vi "GTH.DAC.vi"(6 "FileName":string, 7 "CMD":T1(ring), 8 "Error In":errorcluster, 9 "AMP":u8=1 max=100 step=1, 10 "FREQ":u16, 11 "VISA_USB":refnum<visa-resource-name>) -> (0 "Error Out":errorcluster, 2 "Send CMD":string, 3 "OK?":bool)   [LabVIEW 2012, in "Lib_UEL.ATE.lvlib" / "STM32-CoreBD.lvlib"]
uses:
  STM32-CoreBD.lvlib
  <vilib>/regexp/Match Regular Expression.xnode
panel:
  # "Version History\nV01,2015-2-10, 初始版本."
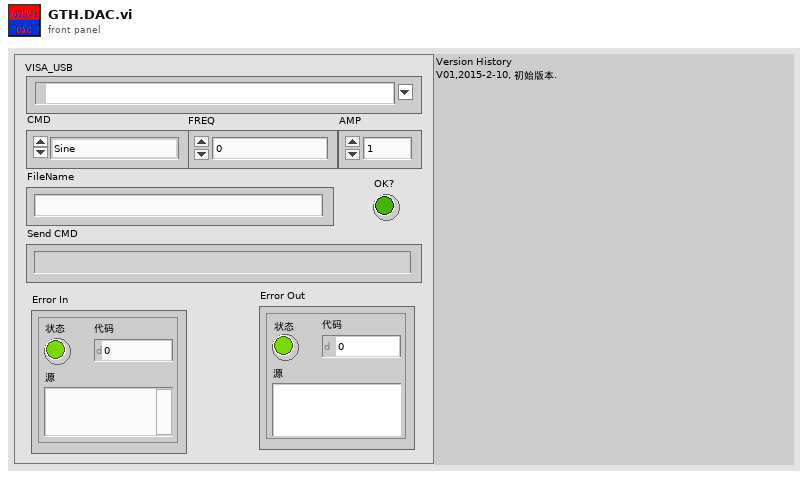
[diagram p1: front panel]
types:
  T1 = enum16{"Sine", "File", "ON_Chip_Pinknoise", "Close Output"}
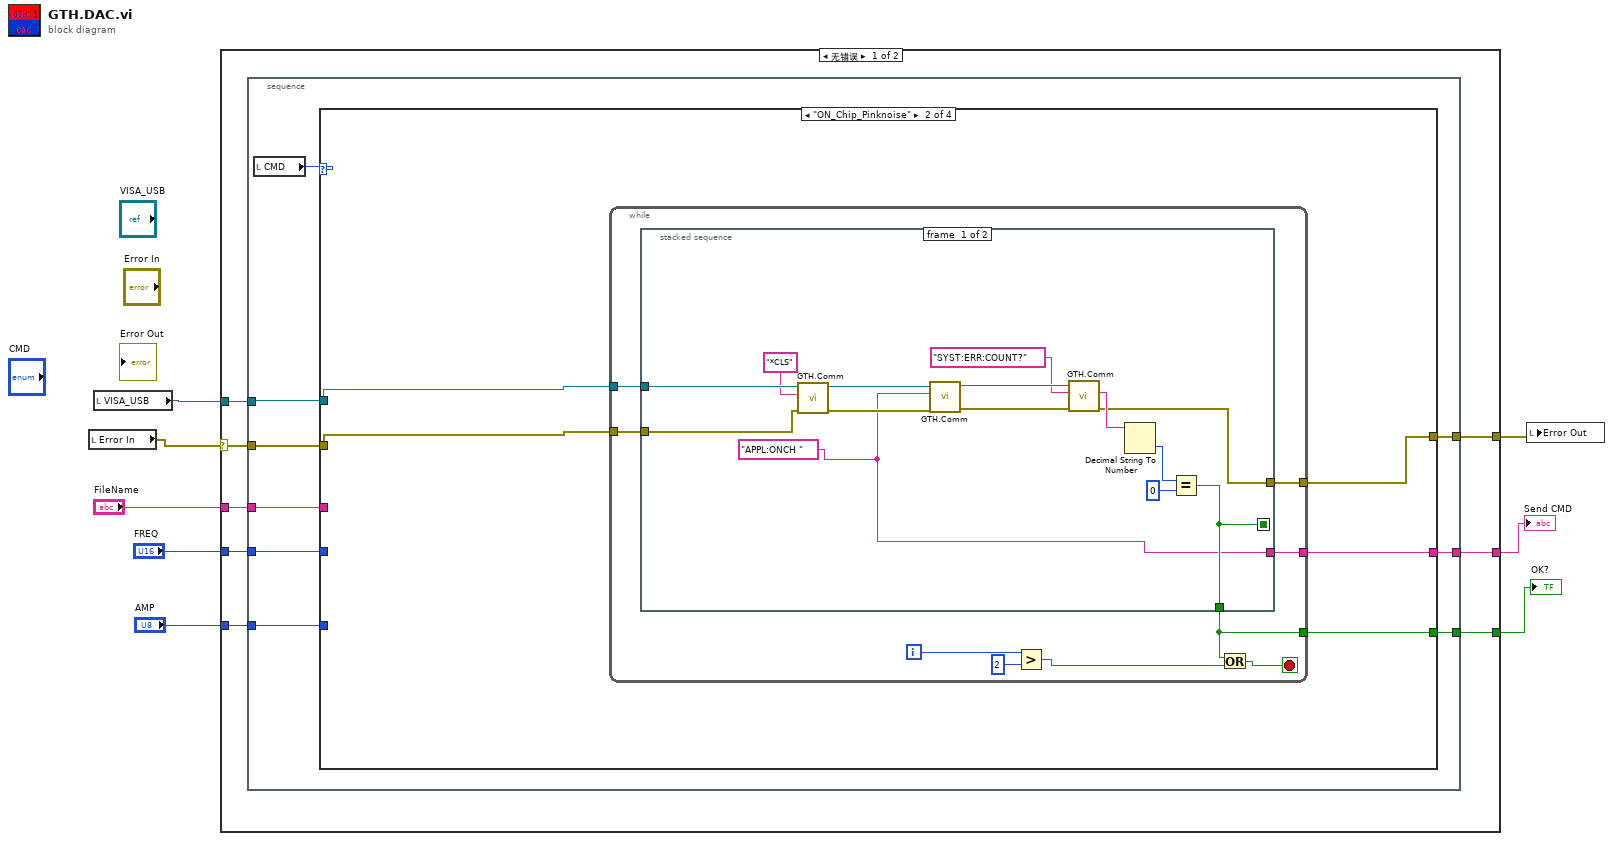
[diagram p0: block diagram]
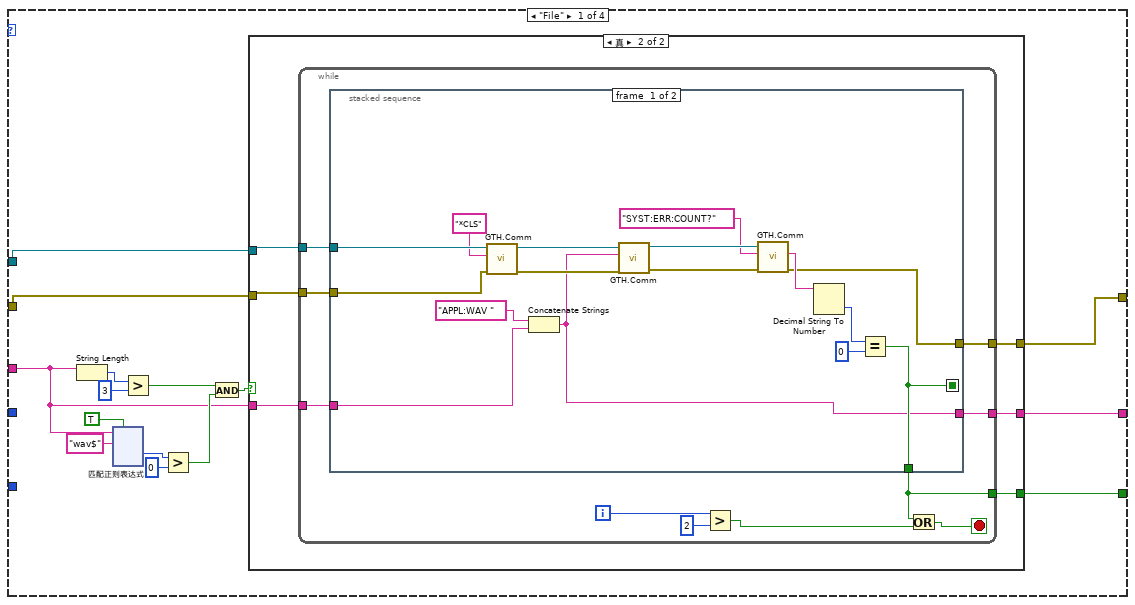
[diagram p2: hidden frame]
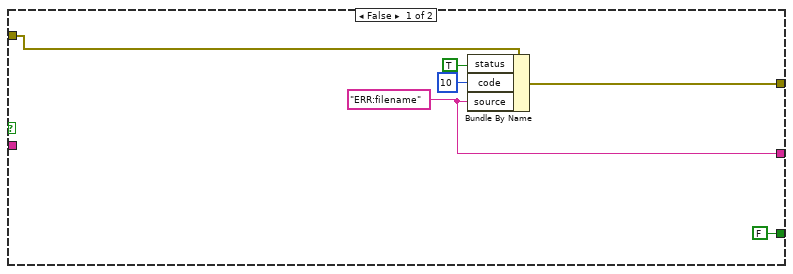
[diagram p3: hidden frame]
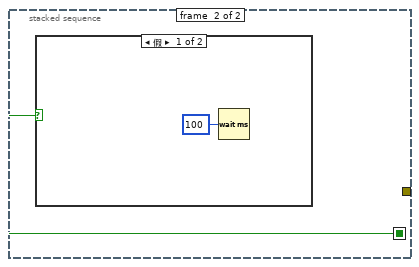
[diagram p4: hidden frame]
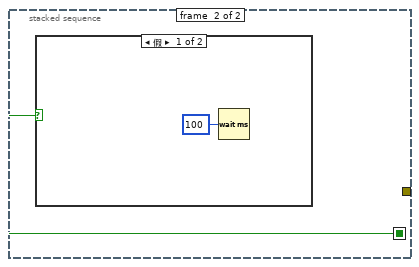
[diagram p6: hidden frame]
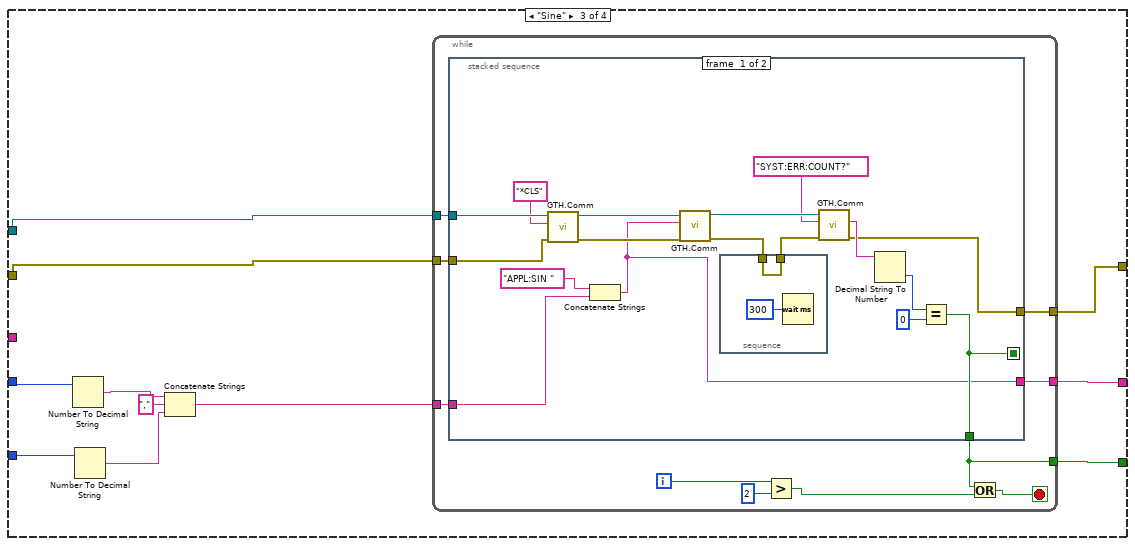
[diagram p8: hidden frame]
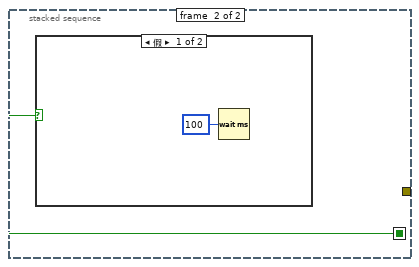
[diagram p9: hidden frame]
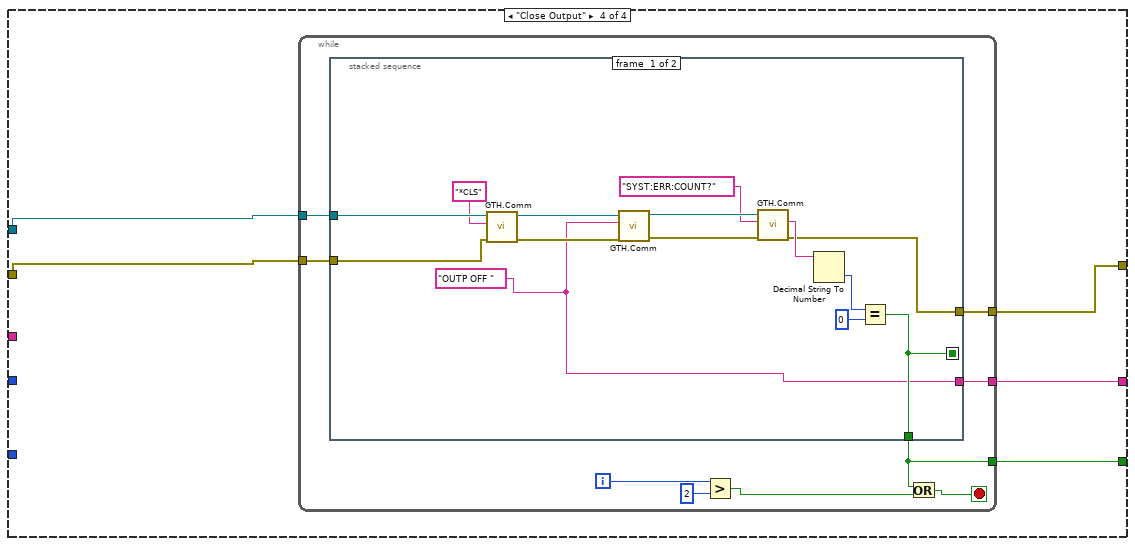
[diagram p11: hidden frame]
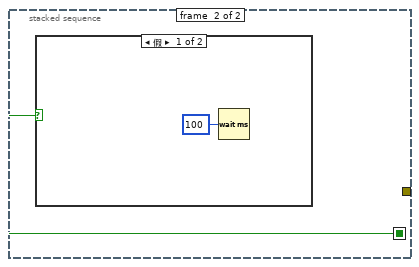
[diagram p12: hidden frame]
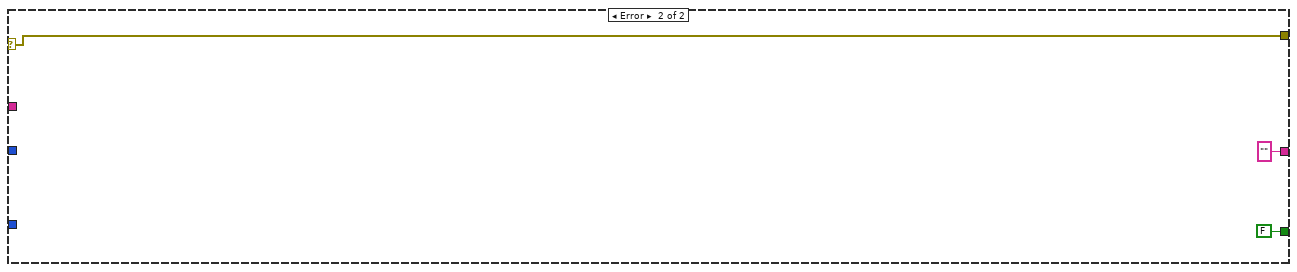
[diagram p14: hidden frame]
diagram:
  n1 = local read "Error In"() -> (w8:errorcluster)
  n2 = local read "VISA_USB"() -> (w6:refnum<visa-resource-name>)
  n3 = case shown="无错误" w8 {
    selector: w8 -> [w16 w296]
    tunnel: [w15 w296] -> w7
    tunnel: w6 -> [w14 _]
    tunnel: "FileName" -> [w13 _]
    tunnel: [w12 "" ("SCPI CMD")] -> w4
    tunnel: [w11 FALSE] -> w3
    tunnel: "FREQ" -> [w10 _]
    tunnel: "AMP" -> [w9 _]
    frame No Error {
      n4 = stacked-sequence {
        tunnel: w16 -> [w23]
        tunnel: [w22] -> w15
        tunnel: w14 -> [w24]
        tunnel: w13 -> [w21]
        tunnel: [w20] -> w12
        tunnel: [w19] -> w11
        tunnel: w10 -> [w18]
        tunnel: w9 -> [w17]
        frame #0 {
          n5 = local read "CMD"() -> (w25:T1)
          n6 = case shown="\"ON_Chip_Pinknoise\"" w25 {
            tunnel: w24 -> [w40 w196 w232 w268]
            tunnel: w23 -> [w39 w195 w231 w267]
            tunnel: [w29 w194 w230 w266] -> w22
            tunnel: w21 -> [w28 _ _ _]
            tunnel: [w27 w193 w229 w265] -> w20
            tunnel: [w26 w192 w228 w264] -> w19
            tunnel: w18 -> [_ _ w227 _]
            tunnel: w17 -> [_ _ w226 _]
            frame "File" {
              n7 = String Length(string=w28) -> (length=w38:i32)
              n8 = xnode "匹配正则表达式"("输入字符串"=w28, "正则表达式"="wav$", "忽略大小写？(F)"=TRUE) -> ("匹配后偏移量"=w34:i32)  [unwired: 3 in, 4 out]
              n9 = Greater?(x=w38, y=3) -> (0:w32:bool)
              n10 = Greater?(x=w34, y=0) -> (0:w31:bool)
              n11 = And(x=w32, y=w31) -> (x .and. y?=w30:bool)
              n12 = case shown="真" w30 {
                tunnel: w40 -> [_ w52]
                tunnel: w39 -> [w46 w51]
                tunnel: [w45 w49] -> w29
                tunnel: w28 -> [_ w50]
                tunnel: [w42 w48] -> w27
                tunnel: [FALSE w47] -> w26
                frame False {
                  w42 = "ERR:filename" ("source")
                  n13 = Bundle By Name(cluster=w46, "status"=TRUE, "code"=10, "source"=w42) -> (w45:errorcluster)
                }
                frame True {
                  n14 = while {
                    tunnel: w52 -> [w62]
                    tunnel: w51 -> [w61]
                    tunnel: w50 -> [w60]
                    tunnel: [w59] -> w49
                    tunnel: [w54] -> w48
                    tunnel: [w53] -> w47
                    i -> [w57]
                    stop <- w58 stop-if-true
                    n15 = stacked-sequence {
                      seq-local: [w64 _] -> [_ w79]
                      tunnel: w62 -> [w78 _]
                      tunnel: w61 -> [w77 _]
                      tunnel: w60 -> [w72 _]
                      tunnel: [w67 _] -> w59
                      tunnel: [w64 _] -> w53
                      tunnel: [w63 _] -> w54
                      frame #0 {
                        n16 = call "GTH.Comm.vi"("Error In"=w77, "SCPI CMD"="*CLS", "USB Port In"=w78) -> ("Error Out"=w74:errorcluster, "USB Port Out"=w75:refnum<visa-resource-name>)  [unwired: 3 in, 4 out]
                        n17 = Concatenate Strings("APPL:WAV " ("SCPI CMD"), w72) -> (w63:string)
                        n18 = call "GTH.Comm.vi"("Error In"=w74, "SCPI CMD"=w63, "USB Port In"=w75) -> ("Error Out"=w70:errorcluster, "USB Port Out"=w71:refnum<visa-resource-name>)  [unwired: 3 in, 4 out]
                        n19 = call "GTH.Comm.vi"("Error In"=w70, "SCPI CMD"="SYST:ERR:COUNT?", "USB Port In"=w71) -> ("Error Out"=w67:errorcluster, "Return"=w68:string)  [unwired: 3 in, 4 out]
                        n20 = Decimal String To Number(string=w68) -> (number=w66:i32)  [unwired: 2 in, 1 out]
                        n21 = Equal?(x=w66, y=0) -> (x = y?=w64:bool)
                      }
                      frame #1 {
                        n22 = case shown="假" w79 {
                          frame False {
                            n23 = Wait (ms)(milliseconds to wait=u32 100 ("等待时间（毫秒）")) -> ()  [unwired: 1 out]
                          }
                          frame True {
                          }
                        }
                      }
                    }
                    n24 = Greater?(x=w57, y=2) -> (0:w55:bool)
                    n25 = Or(x=w53, y=w55) -> (x .or. y?=w58:bool)
                  }
                }
              }
            }
            frame "ON_Chip_Pinknoise" {
              n26 = while {
                tunnel: w196 -> [w205]
                tunnel: w195 -> [w204]
                tunnel: [w203] -> w194
                tunnel: [w198] -> w193
                tunnel: [w197] -> w192
                i -> [w201]
                stop <- w202 stop-if-true
                n27 = stacked-sequence {
                  seq-local: [w207 _] -> [_ w220]
                  tunnel: w205 -> [w219 _]
                  tunnel: w204 -> [w218 _]
                  tunnel: [w210 _] -> w203
                  tunnel: [w207 _] -> w197
                  tunnel: [w206 _] -> w198
                  frame #0 {
                    w206 = "APPL:ONCH " ("SCPI CMD")
                    n28 = call "GTH.Comm.vi"("Error In"=w218, "SCPI CMD"="*CLS", "USB Port In"=w219) -> ("Error Out"=w215:errorcluster, "USB Port Out"=w216:refnum<visa-resource-name>)  [unwired: 3 in, 4 out]
                    n29 = call "GTH.Comm.vi"("Error In"=w215, "SCPI CMD"=w206, "USB Port In"=w216) -> ("Error Out"=w213:errorcluster, "USB Port Out"=w214:refnum<visa-resource-name>)  [unwired: 3 in, 4 out]
                    n30 = call "GTH.Comm.vi"("Error In"=w213, "SCPI CMD"="SYST:ERR:COUNT?", "USB Port In"=w214) -> ("Error Out"=w210:errorcluster, "Return"=w211:string)  [unwired: 3 in, 4 out]
                    n31 = Decimal String To Number(string=w211) -> (number=w209:i32)  [unwired: 2 in, 1 out]
                    n32 = Equal?(x=w209, y=0) -> (x = y?=w207:bool)
                  }
                  frame #1 {
                    n33 = case shown="假" w220 {
                      frame False {
                        n34 = Wait (ms)(milliseconds to wait=u32 100 ("等待时间（毫秒）")) -> ()  [unwired: 1 out]
                      }
                      frame True {
                      }
                    }
                  }
                }
                n35 = Greater?(x=w201, y=2) -> (0:w199:bool)
                n36 = Or(x=w197, y=w199) -> (x .or. y?=w202:bool)
              }
            }
            frame "Sine" {
              n37 = Number To Decimal String(number=w227) -> (decimal integer string=w225:string)  [unwired: 1 in]
              n38 = Number To Decimal String(number=w226) -> (decimal integer string=w224:string)  [unwired: 1 in]
              n39 = Concatenate Strings(w225, "," ("字符串"), w224) -> (w222:string)
              n40 = while {
                tunnel: w232 -> [w242]
                tunnel: w231 -> [w241]
                tunnel: [w240] -> w230
                tunnel: [w235] -> w229
                tunnel: [w234] -> w228
                tunnel: w222 -> [w233]
                i -> [w238]
                stop <- w239 stop-if-true
                n41 = stacked-sequence {
                  seq-local: [w247 _] -> [_ w262]
                  tunnel: w242 -> [w259 _]
                  tunnel: w241 -> [w258 _]
                  tunnel: [w250 _] -> w240
                  tunnel: [w247 _] -> w234
                  tunnel: [w246 _] -> w235
                  tunnel: w233 -> [w245 _]
                  frame #0 {
                    n42 = call "GTH.Comm.vi"("Error In"=w258, "SCPI CMD"="*CLS", "USB Port In"=w259) -> ("Error Out"=w255:errorcluster, "USB Port Out"=w256:refnum<visa-resource-name>)  [unwired: 3 in, 4 out]
                    n43 = Concatenate Strings("APPL:SIN " ("SCPI CMD"), w245) -> (w246:string)
                    n44 = call "GTH.Comm.vi"("Error In"=w255, "SCPI CMD"=w246, "USB Port In"=w256) -> ("Error Out"=w243:errorcluster, "USB Port Out"=w253:refnum<visa-resource-name>)  [unwired: 3 in, 4 out]
                    n45 = stacked-sequence {
                      tunnel: [w261] -> w244
                      tunnel: w243 -> [w261]
                      frame #0 {
                        n46 = Wait (ms)(milliseconds to wait=u32 300 ("等待时间（毫秒）")) -> ()  [unwired: 1 out]
                      }
                    }
                    n47 = call "GTH.Comm.vi"("Error In"=w244, "SCPI CMD"="SYST:ERR:COUNT?", "USB Port In"=w253) -> ("Error Out"=w250:errorcluster, "Return"=w251:string)  [unwired: 3 in, 4 out]
                    n48 = Decimal String To Number(string=w251) -> (number=w249:i32)  [unwired: 2 in, 1 out]
                    n49 = Equal?(x=w249, y=0) -> (x = y?=w247:bool)
                  }
                  frame #1 {
                    n50 = case shown="假" w262 {
                      frame False {
                        n51 = Wait (ms)(milliseconds to wait=u32 100 ("等待时间（毫秒）")) -> ()  [unwired: 1 out]
                      }
                      frame True {
                      }
                    }
                  }
                }
                n52 = Greater?(x=w238, y=2) -> (0:w236:bool)
                n53 = Or(x=w234, y=w236) -> (x .or. y?=w239:bool)
              }
            }
            frame "Close Output" {
              n54 = while {
                tunnel: w268 -> [w277]
                tunnel: w267 -> [w276]
                tunnel: [w275] -> w266
                tunnel: [w270] -> w265
                tunnel: [w269] -> w264
                i -> [w273]
                stop <- w274 stop-if-true
                n55 = stacked-sequence {
                  seq-local: [w279 _] -> [_ w292]
                  tunnel: w277 -> [w291 _]
                  tunnel: w276 -> [w290 _]
                  tunnel: [w282 _] -> w275
                  tunnel: [w279 _] -> w269
                  tunnel: [w278 _] -> w270
                  frame #0 {
                    w278 = "OUTP OFF " ("SCPI CMD")
                    n56 = call "GTH.Comm.vi"("Error In"=w290, "SCPI CMD"="*CLS", "USB Port In"=w291) -> ("Error Out"=w287:errorcluster, "USB Port Out"=w288:refnum<visa-resource-name>)  [unwired: 3 in, 4 out]
                    n57 = call "GTH.Comm.vi"("Error In"=w287, "SCPI CMD"=w278, "USB Port In"=w288) -> ("Error Out"=w285:errorcluster, "USB Port Out"=w286:refnum<visa-resource-name>)  [unwired: 3 in, 4 out]
                    n58 = call "GTH.Comm.vi"("Error In"=w285, "SCPI CMD"="SYST:ERR:COUNT?", "USB Port In"=w286) -> ("Error Out"=w282:errorcluster, "Return"=w283:string)  [unwired: 3 in, 4 out]
                    n59 = Decimal String To Number(string=w283) -> (number=w281:i32)  [unwired: 2 in, 1 out]
                    n60 = Equal?(x=w281, y=0) -> (x = y?=w279:bool)
                  }
                  frame #1 {
                    n61 = case shown="假" w292 {
                      frame False {
                        n62 = Wait (ms)(milliseconds to wait=u32 100 ("等待时间（毫秒）")) -> ()  [unwired: 1 out]
                      }
                      frame True {
                      }
                    }
                  }
                }
                n63 = Greater?(x=w273, y=2) -> (0:w271:bool)
                n64 = Or(x=w269, y=w271) -> (x .or. y?=w274:bool)
              }
            }
          }
        }
      }
    }
    frame Error {
    }
  }
  "Send CMD" <- w4
  "OK?" <- w3
  n65 = local write "Error Out"(w7) -> ()
